vi "NT Read and Format Multiple Entries as String.vi"(8 "error in":errorcluster, 11 "Name Pattern":string) -> (0 "error out":errorcluster, 3 "Formatted Strings":cluster{"Name":string, "Value":string}[](array[cluster]))   [LabVIEW 2020]
doc: "Return the table entries that match the name pattern formatted into strings. Supported wildcards are * and ?."
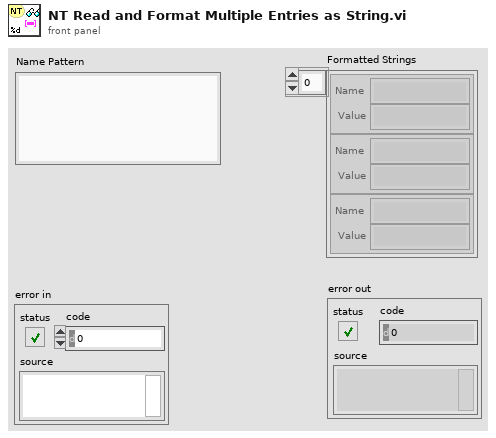
[diagram p1: front panel]
types:
  T1 = typedef "NT Datatype.ctl" = u32
  T2 = cluster{"name":string, "NT_Type":T1, "topicHandle":u32}[]
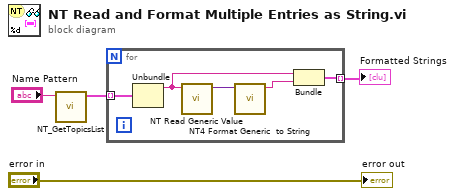
[diagram p0: block diagram]
diagram:
  n1 = call "NT_GetTopicsList.vi"("prefix"="Name Pattern") -> ("Topic List"=w2:T2)  [unwired: 10 in]
  n2 = for {
    tunnel: w2 -> [w9] mode=indexing
    tunnel: [w5] -> w1 mode=indexing
    n3 = Unbundle(w9) -> ("name"=w7:string)  [unwired: 2 out]
    n4 = call "NT Read Generic Value.vi"("name"=w7) -> ("variant value"=w8:variant)  [unwired: 9 in, 1 out]
    n5 = call "NT4 Format Generic  to String.vi"("Variant"=w8) -> ("String"=w6:string)  [unwired: 9 in, 1 out]
    n6 = Bundle("name"=w7, "String"=w6) -> (w5:cluster{"name":string, "String":string})  [unwired: 1 in]
  }
  "Formatted Strings" <- w1
  "error out" <- "error in"
